vi "tmp.vi"() -> ()   [LabVIEW 2016]
uses:
  Motion.lvclass
  Camera/Copy of Controller Folder/Controller.lvclass
panel:
  in  "XYZTheta":dbl[](array[numeric])
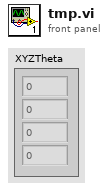
[diagram p1: front panel]
types:
  T1 = typedef "Controller.lvclass/Controllers.ctl" = cluster{"Copy of Motion.lvclass":refnum<class "Motion.lvclass">, "Copy of I-O.lvclass":refnum<class "I-O.lvclass">, "Copy of Dispenser.lvclass":refnum<class "Dispenser.lvclass">}
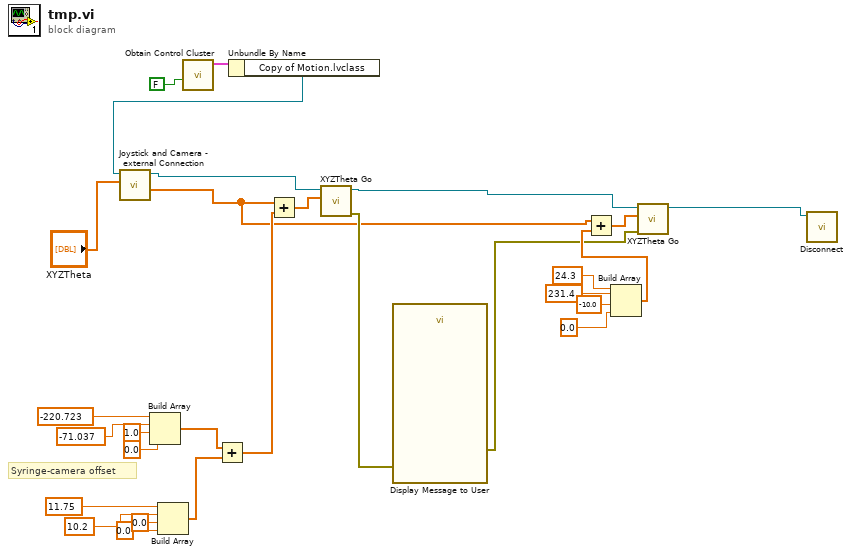
[diagram p0: block diagram]
diagram:
  # "Syringe-camera offset"
  n1 = Build Array(-220.723, -71.037, 1.0 ("element"), 0.0 ("element")) -> (w8:dbl[])
  n2 = Build Array(11.75, 10.2, 0.0 ("element"), 0.0 ("element")) -> (w7:dbl[])
  n3 = call "Obtain Control Cluster.vi"("I/O"=FALSE) -> ("Control Out"=w25:T1)  [unwired: 10 in]
  n4 = Add(x=w8, y=w7) -> (x+y=w2:dbl[])
  n5 = Unbundle By Name(w25) -> ("Copy of Motion.lvclass"=w24:refnum<class "Motion.lvclass">)
  n6 = call "Joystick and Camera - external Connection.vi"("Motion in"=w24, "XYZTheta"="XYZTheta") -> ("Motion out"=w23:refnum<class "Motion.lvclass">, "Gantry"=w1:dbl[])  [unwired: 5 in, 2 out]
  n7 = Add(x=w1, y=w2) -> (x+y=w28:dbl[])
  n8 = call "XYZTheta Go.vi"("XYZTheta In"=w28, "Motion in"=w23) -> ("error out"=w27:errorcluster, "Motion out"=w15:refnum<class "Motion.lvclass">)  [unwired: 7 in, 1 out]
  n9 = call "Display Message to User"("error in (no error)"=w27) -> ("error out"=w13:errorcluster)  [unwired: 9 in, 1 out]
  n10 = Build Array(24.3 ("element"), 231.4 ("element"), -10.0 ("element"), 0.0 ("element")) -> (w18:dbl[])
  n11 = Add(x=w1, y=w18) -> (x+y=w16:dbl[])
  n12 = call "XYZTheta Go.vi"("error in (no error)"=w13, "XYZTheta In"=w16, "Motion in"=w15) -> ("Motion out"=w14:refnum<class "Motion.lvclass">)  [unwired: 6 in, 2 out]
  n13 = call-dynamic "Disconnect.vi"("Controller in"=w14) -> ()  [unwired: 9 in, 1 out]
